vi "FGV_NKT_Param.vi"(3 "error in":errorcluster, 4 "Laser params":T1={"Emission (ON/OFF)"=FALSE, "Wavelength (nm)"=400.0, "Bandwidth (nm)"=10.0, "Power (%)"=0.0, "ND (%)"=0.0} {"ND (%)" min=0.0 max=100.0 step=1.0; "Power (%)" min=0.0 max=100.0 step=1.0; "Wavelength (nm)" min=400.0 max=840.0 step=10.0; "Bandwidth (nm)" min=10.0 max=100.0 step=10.0}, 5 "Action":T2) -> (0 "error out":errorcluster, 1 "Laser params":T1={"Emission (ON/OFF)"=FALSE, "Wavelength (nm)"=400.0, "Bandwidth (nm)"=10.0, "Power (%)"=0.0, "ND (%)"=0.0} {"ND (%)" min=0.0 max=100.0 step=1.0; "Power (%)" min=0.0 max=100.0 step=1.0; "Wavelength (nm)" min=400.0 max=840.0 step=10.0; "Bandwidth (nm)" min=10.0 max=100.0 step=10.0})   [LabVIEW 2026]
uses:
  Controls/TypeDef_FGV.ctl
  Controls/Laser.ctl
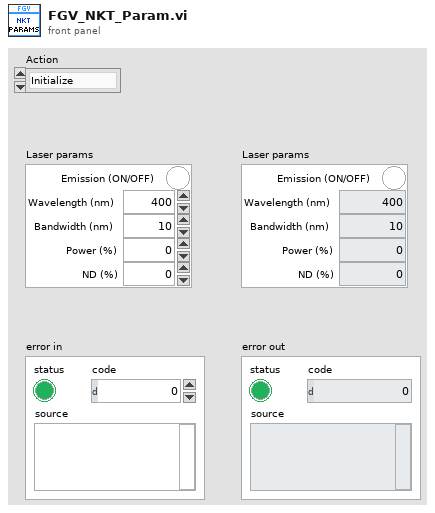
[diagram p1: front panel]
types:
  T1 = typedef "Laser.ctl" = cluster{"Emission (ON/OFF)":bool, "Wavelength (nm)":dbl, "Bandwidth (nm)":dbl, "Power (%)":dbl, "ND (%)":dbl}
  T2 = typedef "TypeDef_FGV.ctl" = enum16{"Initialize", "Write", "Read"}
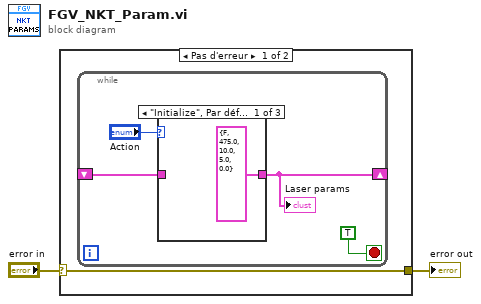
[diagram p0: block diagram]
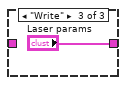
[diagram p3: hidden frame]
diagram:
  n1 = case shown="Pas d'erreur" "error in" {
    selector: "error in" -> [w3 w11]
    tunnel: [w3 w11] -> w2
    frame No Error {
      n2 = while {
        shift-right: [w4] -> _
        shift-left: _ -> [w5]
        stop <- TRUE stop-if-true
        n3 = case shown="\"Initialize\", Par défaut" "Action" {
          tunnel: [T1 {"Emission (ON/OFF)"=FALSE, "Wavelength (nm)"=475.0, "Bandwidth (nm)"=10.0, "Power (%)"=5.0, "ND (%)"=0.0} ("Laser params") w9 "Laser params"] -> w4
          tunnel: w5 -> [_ w9 _]
          frame "Initialize", Default {
          }
          frame "Read" {
          }
          frame "Write" {
          }
        }
        "Laser params" <- w4
      }
    }
    frame Error {
    }
  }
  "error out" <- w2
